vi "theOne.vi"() -> ()   [LabVIEW 2021]
uses:
  <userlib>/er4commlib_labview/er4commlib_labview.lvlib
panel:
  in  "stop":bool
  in  "stop 2":bool
  in  "Boolean":bool
  out "Error String Out":string
  out "error in (no error)":errorcluster
  out "Display 4":dbl[][](graph)
  out "x":dbl
  out "pulseTrainImage":picture
  in  "path to pulseTrainImage file jpg":path=path "C:/neoDiag/MrAnderson/Img/volProtVarAmpl.jpg"
  out "Display 3":dbl[][](graph)=[[0.0, 0.0, 0.0, 0.0, 0.0, 0.0, 0.0, 0.0, 0.0, 0.0, 0.0, 0.0, 0.0, 0.0, 0.0, 0.0, 0.0, 0.0, 0.0, 0.0, 0.0, 0.0, 0.0, 0.0, 0.0, 0.0, 0.0, 0.0, 0.0, 0.0, 0.0, 0.0, 0.0, 0.0, 0.0, 0.0, 0.0, 0.0, 0.0, 0.0, 0.0, 0.0, 0.0, 0.0, 0.0, 0.0, 0.0, 0.0, 0.0, 0.0, 0.0, 0.0, 0.0, 0.0, 0.0, 0.0, 0.0, 0.0, 0.0, 0.0, 0.0, 0.0, 0.0, 0.0, 0.0, 0.0, 0.0, 0.0, 0.0, 0.0, 0.0, 0.0, 0.0, 0.0, 0.0, 0.0, 0.0, 0.0, 0.0, 0.0, 0.0, 0.0, 0.0, 0.0, 0.0, 0.0, 0.0, 0.0, 0.0, 0.0, 0.0, 0.0, 0.0, 0.0, 0.0, 0.0, 0.0, 0.0, 0.0, 0.0, 0.0, 0.0, 0.0, 0.0, 0.0, 0.0, 0.0, 0.0, 0.0, 0.0, 0.0, 0.0, 0.0, 0.0, 0.0, 0.0, 0.0, 0.0, 0.0, 0.0, 0.0, 0.0, 0.0, 0.0, 0.0, 0.0, 0.0, 0.0], [0.004272591326639607, -0.0012207403790398877, -0.008545182653279214, -0.011597033600878933, -0.01281777397991882, -0.013428144169438765, -0.017090365306558428, -0.019531846064638203, -0.01586962492751854, -0.014648884548478652, -0.009765923032319102, -0.007324442274239326, -0.0030518509475997192, 0.004272591326639607, 0.007324442274239326, 0.009765923032319102, 0.013428144169438765, 0.017090365306558428, 0.019531846064638203, 0.02075258644367809, 0.020142216254158147, 0.01770073549607837, 0.014648884548478652, 0.009155552842799158, 0.0061037018951994385, 0.0012207403790398877, -0.003662221137119663, -0.009155552842799158, -0.01098666341135899, -0.01281777397991882, -0.016479995117038484, -0.019531846064638203, -0.017090365306558428, -0.015259254737998596, -0.013428144169438765, -0.00793481246375927, -0.0024414807580797754, 0.0012207403790398877, 0.0061037018951994385, 0.01098666341135899, 0.015259254737998596, 0.016479995117038484, 0.01892147587511826, 0.023194067201757866, 0.02075258644367809, 0.02075258644367809, 0.01586962492751854, 0.01098666341135899, 0.00793481246375927, 0.0012207403790398877, -0.004882961516159551, -0.008545182653279214, -0.01098666341135899, -0.013428144169438765, -0.014648884548478652, -0.018311105685598315, -0.020142216254158147, -0.016479995117038484, -0.013428144169438765, -0.009765923032319102, -0.004882961516159551, -0.0018311105685598315, 0.0030518509475997192, 0.008545182653279214, 0.012207403790398877, 0.01586962492751854, 0.016479995117038484, 0.018311105685598315, 0.020142216254158147, 0.01892147587511826, 0.017090365306558428, 0.013428144169438765, 0.009155552842799158, 0.0061037018951994385, -0.0012207403790398877, -0.0061037018951994385, -0.01098666341135899, -0.014648884548478652, -0.014038514358958708, -0.018311105685598315, -0.020142216254158147, -0.01770073549607837, -0.014648884548478652, -0.012207403790398877, -0.009155552842799158, -0.003662221137119663, 0.0006103701895199438, 0.0061037018951994385, 0.01098666341135899, 0.013428144169438765, 0.015259254737998596, 0.017090365306558428, 0.019531846064638203, 0.018311105685598315, 0.017090365306558428, 0.014648884548478652, 0.009155552842799158, 0.0061037018951994385, 0.0018311105685598315, -0.005493331705679495, -0.008545182653279214, -0.012207403790398877, -0.012207403790398877, -0.014648884548478652, -0.018311105685598315, -0.017090365306558428, -0.016479995117038484, -0.01281777397991882, -0.00793481246375927, -0.005493331705679495, -0.0012207403790398877, 0.0061037018951994385, 0.01098666341135899, 0.014038514358958708, 0.01586962492751854, 0.016479995117038484, 0.019531846064638203, 0.020142216254158147, 0.018311105685598315, 0.014648884548478652, 0.014648884548478652, 0.009155552842799158, 0.003662221137119663, -0.0018311105685598315, -0.00793481246375927, -0.010376293221839045, -0.013428144169438765, -0.015259254737998596], [0.0012207403790398877, -0.003662221137119663, -0.008545182653279214, -0.011597033600878933, -0.014038514358958708, -0.014648884548478652, -0.016479995117038484, -0.01770073549607837, -0.015259254737998596, -0.013428144169438765, -0.011597033600878933, -0.008545182653279214, -0.004882961516159551, 0.0006103701895199438, 0.005493331705679495, 0.007324442274239326, 0.008545182653279214, 0.009765923032319102, 0.012207403790398877, 0.014038514358958708, 0.01281777397991882, 0.01098666341135899, 0.00793481246375927, 0.004882961516159551, 0.0024414807580797754, -0.0024414807580797754, -0.0061037018951994385, -0.010376293221839045, -0.011597033600878933, -0.013428144169438765, -0.014648884548478652, -0.017090365306558428, -0.01586962492751854, -0.014038514358958708, -0.01281777397991882, -0.00793481246375927, -0.005493331705679495, -0.0030518509475997192, 0.0030518509475997192, 0.007324442274239326, 0.009155552842799158, 0.010376293221839045, 0.012207403790398877, 0.015259254737998596, 0.014038514358958708, 0.012207403790398877, 0.009765923032319102, 0.0061037018951994385, 0.0030518509475997192, 0.0006103701895199438, -0.005493331705679495, -0.009155552842799158, -0.01098666341135899, -0.014038514358958708, -0.014038514358958708, -0.017090365306558428, -0.01586962492751854, -0.01586962492751854, -0.012207403790398877, -0.010376293221839045, -0.00793481246375927, -0.004272591326639607, 0.0018311105685598315, 0.005493331705679495, 0.007324442274239326, 0.010376293221839045, 0.012207403790398877, 0.01281777397991882, 0.014648884548478652, 0.013428144169438765, 0.01098666341135899, 0.008545182653279214, 0.005493331705679495, 0.003662221137119663, -0.0030518509475997192, -0.006714072084719382, -0.008545182653279214, -0.01281777397991882, -0.014648884548478652, -0.01586962492751854, -0.01586962492751854, -0.015259254737998596, -0.014648884548478652, -0.01098666341135899, -0.007324442274239326, -0.003662221137119663, -0.0012207403790398877, 0.0024414807580797754, 0.0061037018951994385, 0.009765923032319102, 0.009765923032319102, 0.012207403790398877, 0.015259254737998596, 0.014648884548478652, 0.01098666341135899, 0.009155552842799158, 0.007324442274239326, 0.003662221137119663, 0.0, -0.004882961516159551, -0.009155552842799158, -0.011597033600878933, -0.013428144169438765, -0.014648884548478652, -0.01586962492751854, -0.017090365306558428, -0.016479995117038484, -0.014648884548478652, -0.008545182653279214, -0.005493331705679495, -0.0030518509475997192, 0.0018311105685598315, 0.004882961516159551, 0.008545182653279214, 0.010376293221839045, 0.011597033600878933, 0.014038514358958708, 0.014648884548478652, 0.01281777397991882, 0.009765923032319102, 0.009155552842799158, 0.0061037018951994385, 0.0024414807580797754, -0.0030518509475997192, -0.0061037018951994385, -0.010376293221839045, -0.012207403790398877, -0.012207403790398877], [-0.0061037018951994385, -0.012207403790398877, -0.015259254737998596, -0.018311105685598315, -0.022583697012237922, -0.022583697012237922, -0.023194067201757866, -0.02380443739127781, -0.02380443739127781, -0.022583697012237922, -0.02075258644367809, -0.016479995117038484, -0.013428144169438765, -0.007324442274239326, -0.0024414807580797754, 0.0, 0.0012207403790398877, 0.0012207403790398877, 0.004882961516159551, 0.006714072084719382, 0.003662221137119663, 0.0024414807580797754, 0.0006103701895199438, -0.0018311105685598315, -0.004882961516159551, -0.009155552842799158, -0.014038514358958708, -0.018311105685598315, -0.021362956633198035, -0.022583697012237922, -0.02380443739127781, -0.02685628833887753, -0.02685628833887753, -0.024414807580797754, -0.02197332682271798, -0.017090365306558428, -0.012207403790398877, -0.009155552842799158, -0.003662221137119663, 0.0, 0.0030518509475997192, 0.0030518509475997192, 0.003662221137119663, 0.006714072084719382, 0.006714072084719382, 0.003662221137119663, 0.0030518509475997192, 0.0, -0.003662221137119663, -0.007324442274239326, -0.011597033600878933, -0.015259254737998596, -0.017090365306558428, -0.020142216254158147, -0.021362956633198035, -0.024414807580797754, -0.024414807580797754, -0.023194067201757866, -0.02075258644367809, -0.018311105685598315, -0.01586962492751854, -0.01281777397991882, -0.006714072084719382, -0.0030518509475997192, 0.0006103701895199438, 0.0030518509475997192, 0.0030518509475997192, 0.005493331705679495, 0.0061037018951994385, 0.003662221137119663, 0.003662221137119663, 0.0030518509475997192, -0.0024414807580797754, -0.004882961516159551, -0.009155552842799158, -0.016479995117038484, -0.01892147587511826, -0.02075258644367809, -0.02197332682271798, -0.02380443739127781, -0.026245918149357585, -0.02380443739127781, -0.024414807580797754, -0.02197332682271798, -0.017090365306558428, -0.014038514358958708, -0.008545182653279214, -0.004272591326639607, -0.0012207403790398877, 0.0030518509475997192, 0.003662221137119663, 0.004882961516159551, 0.007324442274239326, 0.0061037018951994385, 0.003662221137119663, 0.0012207403790398877, -0.0012207403790398877, -0.004272591326639607, -0.00793481246375927, -0.01281777397991882, -0.01770073549607837, -0.019531846064638203, -0.020142216254158147, -0.022583697012237922, -0.026245918149357585, -0.024414807580797754, -0.02380443739127781, -0.02197332682271798, -0.01770073549607837, -0.014648884548478652, -0.01281777397991882, -0.0061037018951994385, 0.0006103701895199438, 0.0012207403790398877, 0.0030518509475997192, 0.003662221137119663, 0.006714072084719382, 0.004882961516159551, 0.004882961516159551, 0.0024414807580797754, 0.0, -0.003662221137119663, -0.00793481246375927, -0.012207403790398877, -0.016479995117038484, -0.02075258644367809, -0.021362956633198035, -0.022583697012237922], [-0.004882961516159551, -0.011597033600878933, -0.015259254737998596, -0.01770073549607837, -0.02197332682271798, -0.023194067201757866, -0.026245918149357585, -0.028077028717917417, -0.02685628833887753, -0.02380443739127781, -0.020142216254158147, -0.015259254737998596, -0.010376293221839045, -0.005493331705679495, 0.0024414807580797754, 0.004882961516159551, 0.009155552842799158, 0.009765923032319102, 0.013428144169438765, 0.015259254737998596, 0.012207403790398877, 0.010376293221839045, 0.006714072084719382, 0.0018311105685598315, -0.0012207403790398877, -0.007324442274239326, -0.014648884548478652, -0.01770073549607837, -0.02075258644367809, -0.02075258644367809, -0.02563554795983764, -0.028077028717917417, -0.02563554795983764, -0.025025177770317698, -0.02075258644367809, -0.017090365306558428, -0.01281777397991882, -0.00793481246375927, -0.0018311105685598315, 0.003662221137119663, 0.0061037018951994385, 0.009155552842799158, 0.010376293221839045, 0.01281777397991882, 0.01281777397991882, 0.010376293221839045, 0.007324442274239326, 0.003662221137119663, -0.0006103701895199438, -0.003662221137119663, -0.014038514358958708, -0.01770073549607837, -0.019531846064638203, -0.024414807580797754, -0.024414807580797754, -0.028077028717917417, -0.028077028717917417, -0.02685628833887753, -0.023194067201757866, -0.01892147587511826, -0.015259254737998596, -0.011597033600878933, -0.0030518509475997192, 0.0012207403790398877, 0.003662221137119663, 0.00793481246375927, 0.009155552842799158, 0.013428144169438765, 0.014038514358958708, 0.011597033600878933, 0.00793481246375927, 0.0061037018951994385, 0.0012207403790398877, -0.0018311105685598315, -0.006714072084719382, -0.013428144169438765, -0.017090365306558428, -0.022583697012237922, -0.023194067201757866, -0.02563554795983764, -0.02868739890743736, -0.024414807580797754, -0.022583697012237922, -0.020142216254158147, -0.014648884548478652, -0.014038514358958708, -0.006714072084719382, 0.0, 0.003662221137119663, 0.0061037018951994385, 0.008545182653279214, 0.012207403790398877, 0.014038514358958708, 0.013428144169438765, 0.012207403790398877, 0.00793481246375927, 0.003662221137119663, -0.0006103701895199438, -0.005493331705679495, -0.012207403790398877, -0.018311105685598315, -0.021362956633198035, -0.023194067201757866, -0.02685628833887753, -0.02868739890743736, -0.027466658528397473, -0.02563554795983764, -0.022583697012237922, -0.018311105685598315, -0.014038514358958708, -0.010376293221839045, -0.003662221137119663, 0.0024414807580797754, 0.005493331705679495, 0.00793481246375927, 0.008545182653279214, 0.013428144169438765, 0.01281777397991882, 0.01098666341135899, 0.01098666341135899, 0.005493331705679495, 0.0006103701895199438, -0.0018311105685598315, -0.009765923032319102, -0.01586962492751854, -0.01892147587511826, -0.02197332682271798, -0.02197332682271798], [0.0, 0.0, 0.0, 0.0, 0.0, 0.0, 0.0, 0.0, 0.0, 0.0, 0.0, 0.0, 0.0, 0.0, 0.0, 0.0, 0.0, 0.0, 0.0, 0.0, 0.0, 0.0, 0.0, 0.0, 0.0, 0.0, 0.0, 0.0, 0.0, 0.0, 0.0, 0.0, 0.0, 0.0, 0.0, 0.0, 0.0, 0.0, 0.0, 0.0, 0.0, 0.0, 0.0, 0.0, 0.0, 0.0, 0.0, 0.0, 0.0, 0.0, 0.0, 0.0, 0.0, 0.0, 0.0, 0.0, 0.0, 0.0, 0.0, 0.0, 0.0, 0.0, 0.0, 0.0, 0.0, 0.0, 0.0, 0.0, 0.0, 0.0, 0.0, 0.0, 0.0, 0.0, 0.0, 0.0, 0.0, 0.0, 0.0, 0.0, 0.0, 0.0, 0.0, 0.0, 0.0, 0.0, 0.0, 0.0, 0.0, 0.0, 0.0, 0.0, 0.0, 0.0, 0.0, 0.0, 0.0, 0.0, 0.0, 0.0, 0.0, 0.0, 0.0, 0.0, 0.0, 0.0, 0.0, 0.0, 0.0, 0.0, 0.0, 0.0, 0.0, 0.0, 0.0, 0.0, 0.0, 0.0, 0.0, 0.0, 0.0, 0.0, 0.0, 0.0, 0.0, 0.0, 0.0, 0.0]]
  out "counterArraySize":i32=2500
  out "runningCounterFlag":bool=TRUE
  out "runningCounter":i32=1488
  out "initialized array":dbl[][](array[numeric])
  out "function return":u32(ring)
  in  "Tab Control":enum32{"AcqPara", "AdvPara"}(tab)
  in  "Acquisition Parameters":T1={"Camera "=FALSE, "Voltage stimulus"=FALSE, "Period [ms]"=200.0, "Duration [ms]"=0.2, "Delay [ms]"=0.0, "Pulses [#]"=10, "Vhold [mV]"=-50.0, "Vpulse [mV]"=0.0, "Vstep [mV]"=10.0, "N"=10, "Thold [ms]"=0.0, "Tpulse [ms]"=200.0, "sampling rate [kHz]"="1,25", "current range [nA]"="20", "time [s]"=2.0} {"Tpulse [ms]" format="%_5f"; "Thold [ms]" format="%_5f"; "Vstep [mV]" format="%_5f"; "Vpulse [mV]" format="%_5f"; "Vhold [mV]" format="%_5f"; "Delay [ms]" format="%_5f"; "Duration [ms]" format="%_5f"; "Period [ms]" format="%_5f"}
  in  "advancedSettings":T2={"Channels to read"=6, "update rate of main loop"=100}
  out "Error Out Int":u32
  out "Error Out String":string
  out "E4 parameters":T3={"currentChannelsNum out"=1, "voltageChannelsNum out"=4, "gpChannelsNum out"=1, "sampling rate [kHz]"=1.25, "real sampling rate [kHz]"=1.220703125, "Ch_min"=-20.0, "Ch_max"=20.0, "Ch_step"=0.0006103701895199438, "Ch_unit"=1e-09}
  in  "Display 1":cluster{"ChArray":bool[]}={"ChArray"=[FALSE, TRUE, TRUE, TRUE, FALSE, FALSE]}
  out "Display 2":dbl[][](graph)
  in  "Live":bool
  out "status out":T4={"availableDataPackets"=128, "bufferOverflowFlag"=FALSE, "lostDataFlag"=FALSE, "saturationFlag"=FALSE, "currentRangeIncreaseFlag"=FALSE, "currentRangeDecreaseFlag"=TRUE, "communicationErrorFlag"=FALSE}
  out "Error Read":errorcluster
  # "DataCh1"
  # "DataCh2"
  # "DataCh3"
  # "DataCh4"
  # "Voltage"
  # "Trigger"
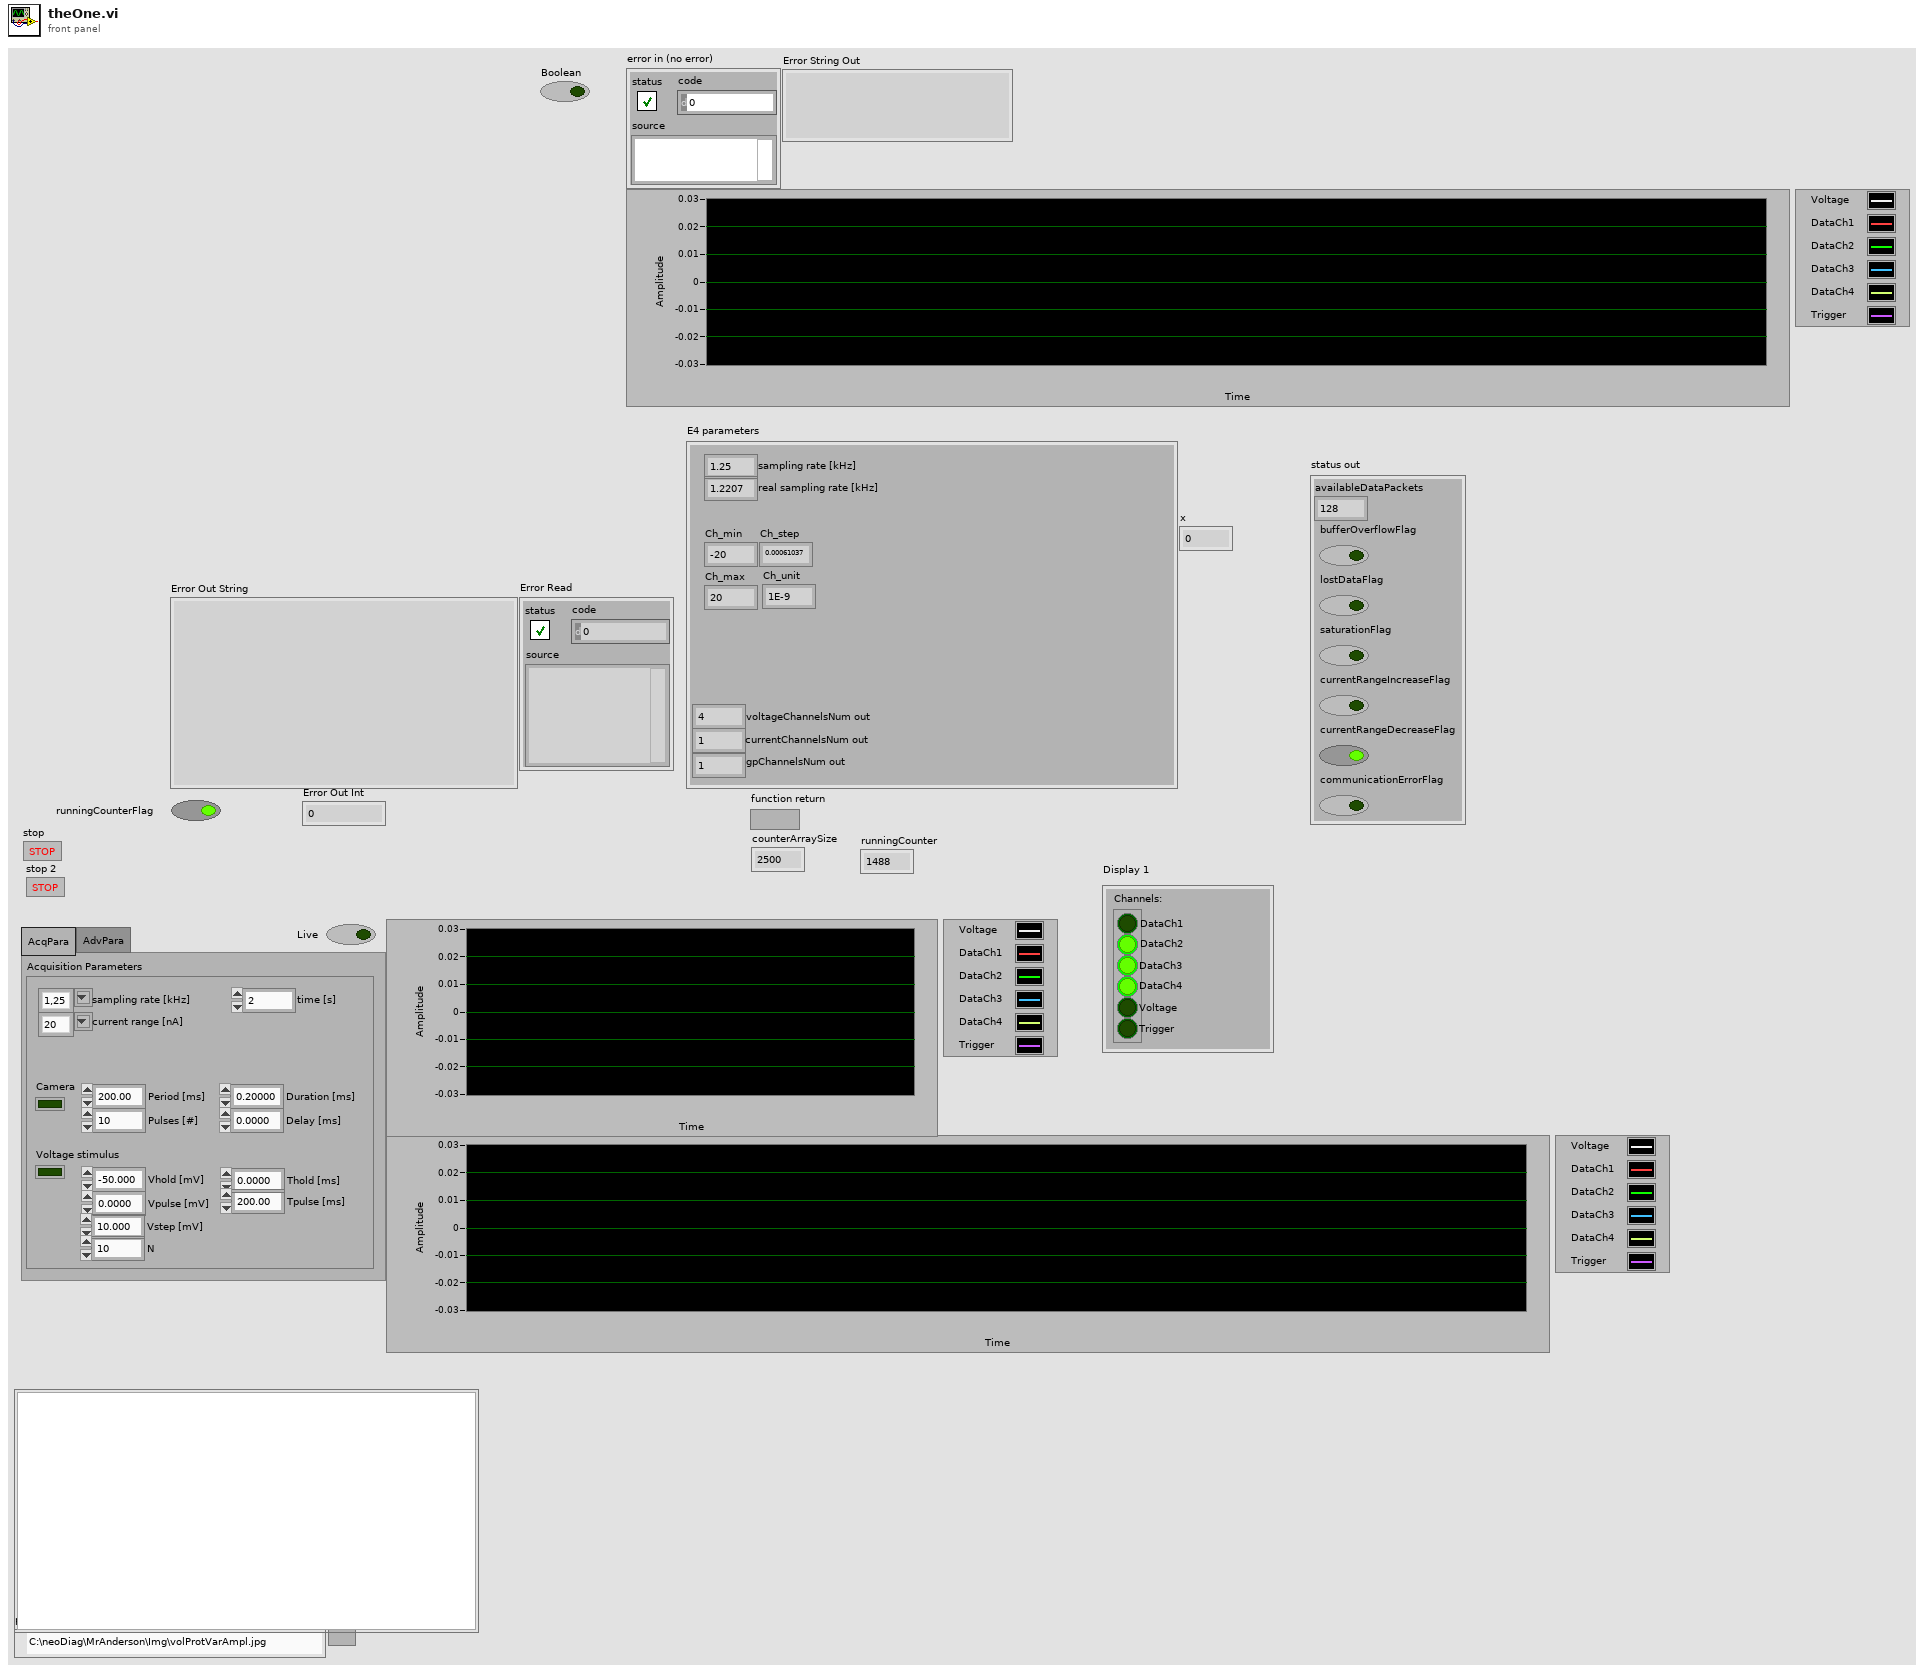
[diagram p1: front panel]
types:
  T1 = cluster{"Camera ":bool, "Voltage stimulus":bool, "Period [ms]":dbl, "Duration [ms]":dbl, "Delay [ms]":dbl, "Pulses [#]":u32, "Vhold [mV]":dbl, "Vpulse [mV]":dbl, "Vstep [mV]":dbl, "N":u32, "Thold [ms]":dbl, "Tpulse [ms]":dbl, "sampling rate [kHz]":string, "current range [nA]":string, "time [s]":dbl}
  T2 = cluster{"Channels to read":i32, "update rate of main loop":i32}
  T3 = cluster{"currentChannelsNum out":u32, "voltageChannelsNum out":u32, "gpChannelsNum out":u32, "sampling rate [kHz]":dbl, "real sampling rate [kHz]":dbl, "Ch_min":dbl, "Ch_max":dbl, "Ch_step":dbl, "Ch_unit":dbl}
  T4 = cluster{"availableDataPackets":u32, "bufferOverflowFlag":bool, "lostDataFlag":bool, "saturationFlag":bool, "currentRangeIncreaseFlag":bool, "currentRangeDecreaseFlag":bool, "communicationErrorFlag":bool}
  T5 = typedef "imagedata.ctl" = cluster{"image type":i32, "image depth":i32, "image":u8[], "mask":u8[], "colors":u32[], "Rectangle":cluster{"left":i16, "top":i16, "right":i16, "bottom":i16}}
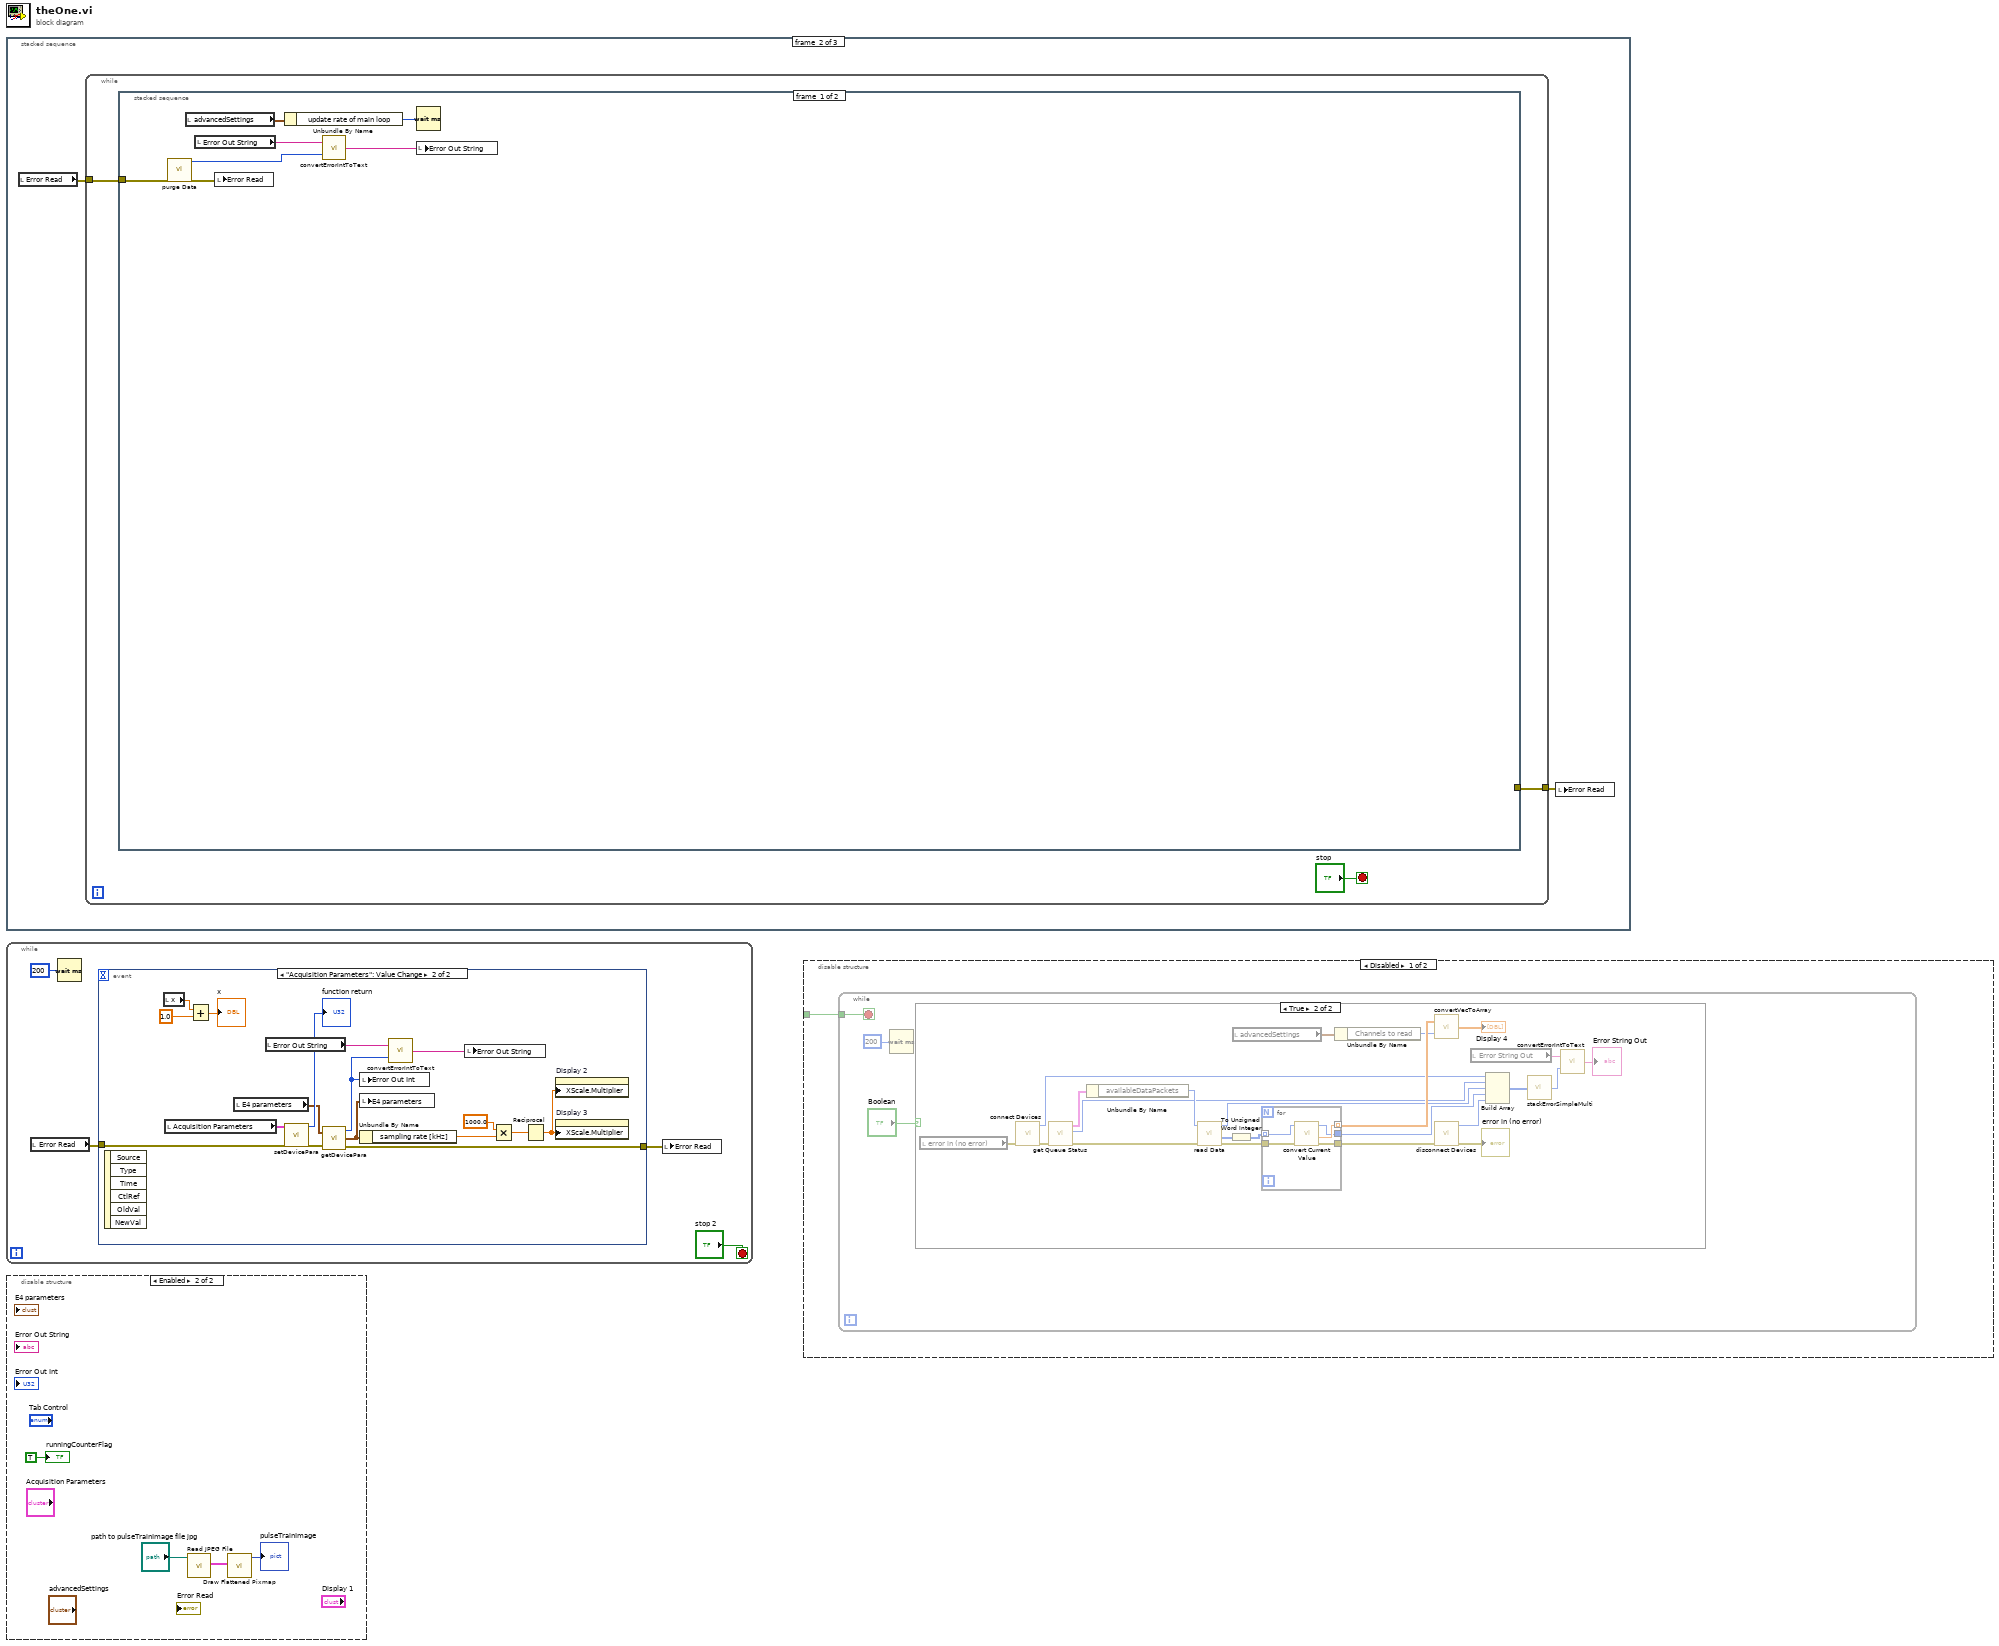
[diagram p0: block diagram]
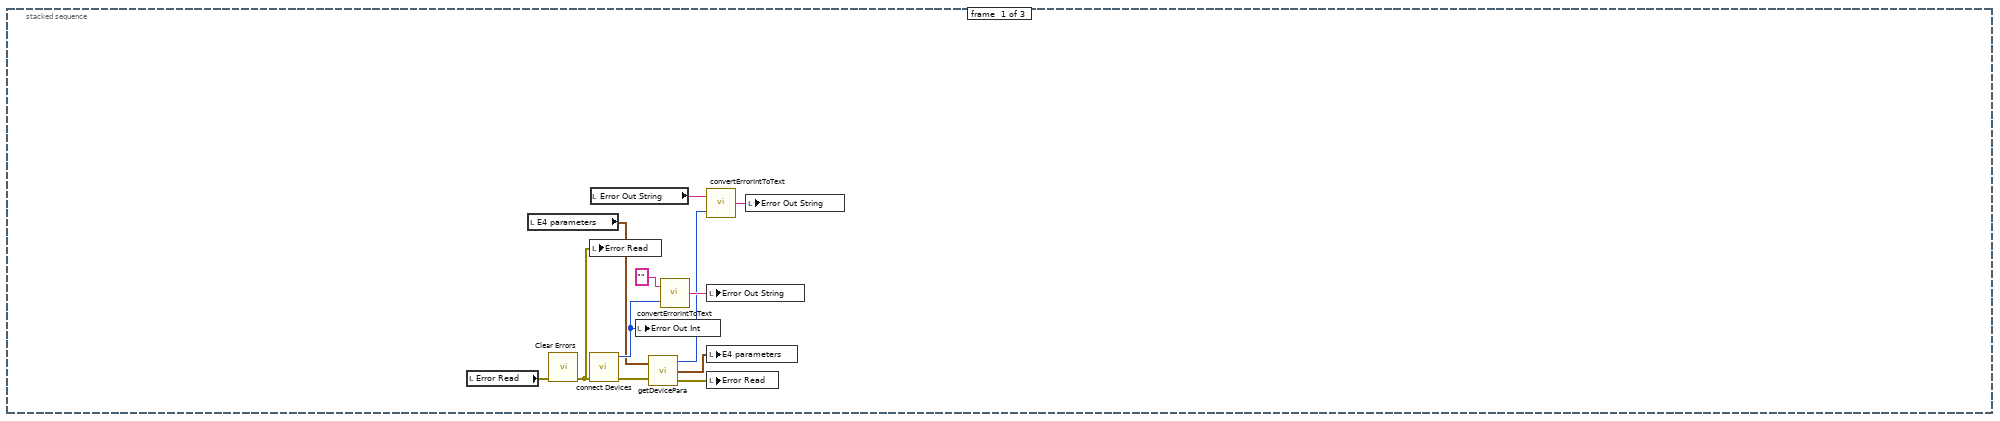
[diagram p4: hidden frame]
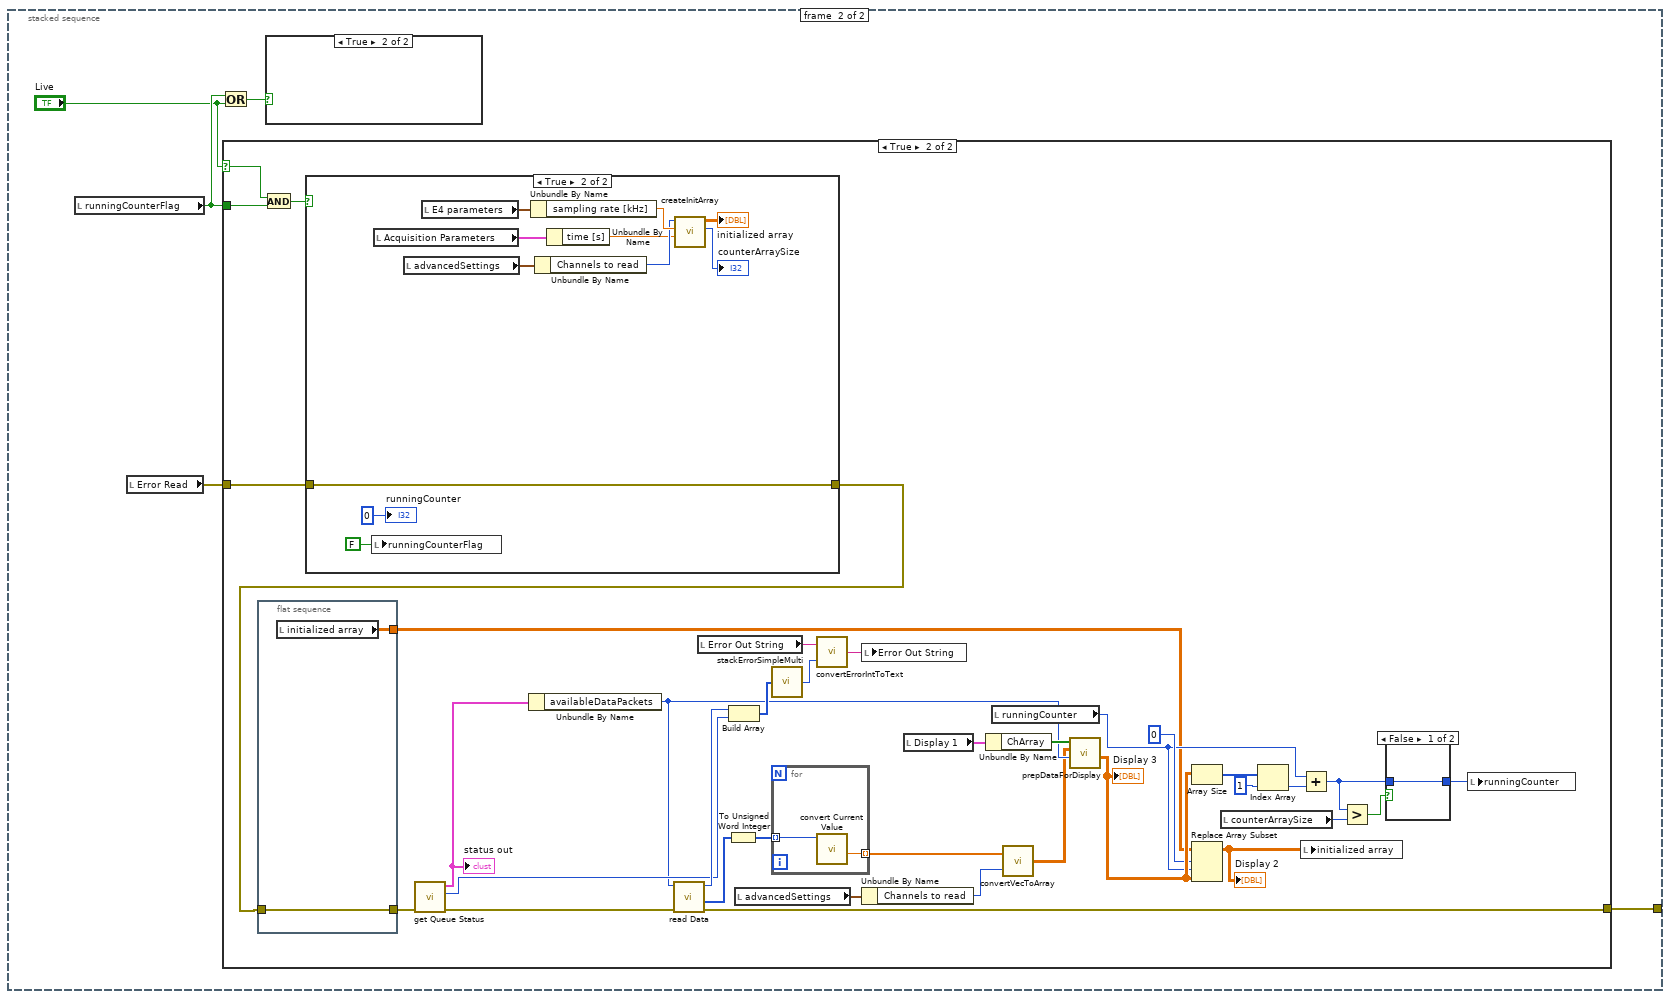
[diagram p5: hidden frame]
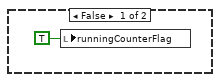
[diagram p6: hidden frame]
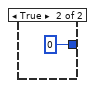
[diagram p9: hidden frame]
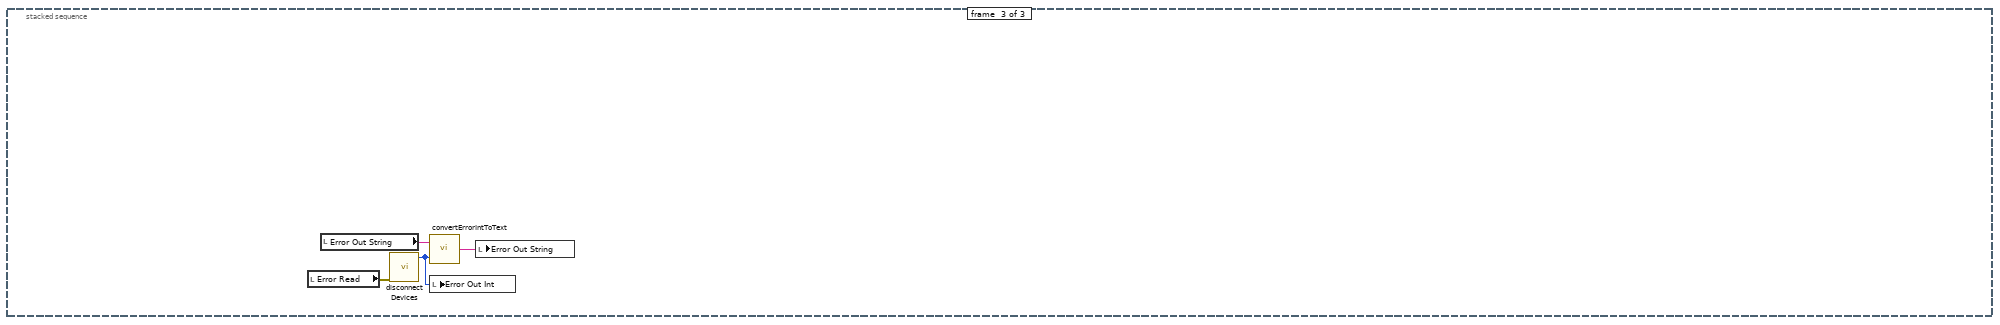
[diagram p10: hidden frame]
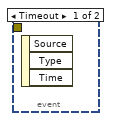
[diagram p11: hidden frame]
diagram:
  n1 = stacked-sequence {
    frame #0 {
      n2 = local read "Error Read"() -> (w3:errorcluster)
      n3 = local read "E4 parameters"() -> (w8:T3)
      n4 = call <vilib>:"Clear Errors.vi"("error in (no error)"=w3) -> ("error out"=w2:errorcluster)  [unwired: 5 in, 1 out]
      n5 = local write "Error Read"(w2) -> ()
      n6 = call <userlib>:"connect Devices.vi"("error in (no error)"=w2) -> ("error out"=w9:errorcluster, "function return"=w12:u32)  [unwired: 9 in]
      n7 = local read "Error Out String"() -> (w5:string)
      n8 = local write "Error Out Int"(w12) -> ()
      n9 = call "getDevicePara.vi"("Seetings in"=w8, "error in (no error)"=w9) -> ("Error Out"=w6:u32, "Seetings out"=w7:T3, "error out"=w1:errorcluster)
      n10 = call "convertErrorIntToText.vi"("Error Int In (function return)"=w12, "Error String In"="" ("String 2")) -> ("Error String Out"=w11:string)
      n11 = call "convertErrorIntToText.vi"("Error Int In (function return)"=w6, "Error String In"=w5) -> ("Error String Out"=w4:string)
      n12 = local write "Error Out String"(w11) -> ()
      n13 = local write "E4 parameters"(w7) -> ()
      n14 = local write "Error Read"(w1) -> ()
      n15 = local write "Error Out String"(w4) -> ()
    }
    frame #1 {
      n16 = local read "Error Read"() -> (w13:errorcluster)
      n17 = while {
        tunnel: w13 -> [w16]
        tunnel: [w17] -> w14
        stop <- "stop" stop-if-true
        n18 = stacked-sequence {
          tunnel: w16 -> [w24 _]
          tunnel: [_ w29] -> w17
          frame #0 {
            n19 = call <userlib>:"purge Data.vi"("error in (no error)"=w24) -> ("error out"=w18:errorcluster, "function return"=w22:u32)  [unwired: 9 in]
            n20 = local read "advancedSettings"() -> (w20:T2)
            n21 = local read "Error Out String"() -> (w23:string)
            n22 = local write "Error Read"(w18) -> ()
            n23 = Unbundle By Name(w20) -> ("update rate of main loop"=w19:i32)
            n24 = call "convertErrorIntToText.vi"("Error Int In (function return)"=w22, "Error String In"=w23) -> ("Error String Out"=w21:string)
            n25 = Wait (ms)(milliseconds to wait=w19) -> ()  [unwired: 1 out]
            n26 = local write "Error Out String"(w21) -> ()
          }
          frame #1 {
            n27 = local read "runningCounterFlag"() -> (w28:bool)
            n28 = local read "Error Read"() -> (w25:errorcluster)
            n29 = Or(x=w28, y="Live") -> (x .or. y?=w26:bool)
            n30 = case shown="True" "Live" {
              selector: "Live" -> [_ w45]
              tunnel: w25 -> [w31 w41]
              tunnel: [w31 w65] -> w29
              tunnel: w28 -> [_ w44]
              frame False {
              }
              frame True {
                n31 = flat-sequence {
                  tunnel: w32 -> [w69]
                  tunnel: [w69] -> w34
                  tunnel: [w68] -> w35
                  frame #0 {
                    n32 = local read "initialized array"() -> (w68:dbl[][])
                  }
                }
                n33 = And(x=w45, y=w44) -> (x .and. y?=w43:bool)
                n34 = case shown="True" w43 {
                  tunnel: w41 -> [w70 w73]
                  tunnel: [w70 w73] -> w32
                  frame False {
                  }
                  frame True {
                    n35 = local write "runningCounterFlag"(FALSE ("runningCounterFlag")) -> ()
                    n36 = local read "Acquisition Parameters"() -> (w72:T1)
                    n37 = local read "advancedSettings"() -> (w76:T2)
                    n38 = local read "E4 parameters"() -> (w78:T3)
                    n39 = Unbundle By Name(w78) -> ("sampling rate [kHz]"=w79:dbl)
                    n40 = Unbundle By Name(w76) -> ("Channels to read"=w77:i32)
                    n41 = Unbundle By Name(w72) -> ("time [s]"=w71:dbl)
                    n42 = call "createInitArray.vi"("timeAxisLim"=w71, "sampling rate [kHz]"=w79, "Channels to read"=w77) -> ("Numeric"=→"counterArraySize":i32, "Array"=→"initialized array":dbl[][])  [unwired: 7 in]
                    "runningCounter" <- 0 ("runningCounter")
                  }
                }
                n43 = call <userlib>:"get Queue Status.vi"("error in (no error)"=w34) -> ("error out"=w66:errorcluster, "function return"=w63:u32, "status out"=w67:T4)  [unwired: 8 in]
                "status out" <- w67
                n44 = Unbundle By Name(w67) -> ("availableDataPackets"=w55:u32)
                n45 = call <userlib>:"read Data.vi"("error in (no error)"=w66, "dataToRead"=w55) -> ("error out"=w65:errorcluster, "buffer out"=w33:i16[], "function return"=w64:u32)  [unwired: 6 in, 1 out]
                n46 = local read "Error Out String"() -> (w59:string)
                n47 = To Unsigned Word Integer(number=w33) -> (unsigned 16bit integer=w54:u16[])
                n48 = Build Array(w64, w63) -> (w62:u32[])
                n49 = local read "advancedSettings"() -> (w56:T2)
                n50 = call "stackErrorSimpleMulti.vi"("Error List"=w62) -> ("Error Out"=w61:u32)
                n51 = for {
                  tunnel: w54 -> [w85] mode=indexing
                  tunnel: [w84] -> w53 mode=indexing
                  n52 = call <userlib>:"convert Current Value.vi"("intValue"=w85) -> ("fltValue out"=w84:dbl)  [unwired: 8 in, 2 out]
                }
                n53 = call "convertErrorIntToText.vi"("Error Int In (function return)"=w61, "Error String In"=w59) -> ("Error String Out"=w60:string)
                n54 = local write "Error Out String"(w60) -> ()
                n55 = Unbundle By Name(w56) -> ("Channels to read"=w52:i32)
                n56 = local read "Display 1"() -> (w58:cluster{"ChArray":bool[]})
                n57 = Unbundle By Name(w58) -> ("ChArray"=w57:bool[])
                n58 = local read "runningCounter"() -> (w37:i32)
                n59 = call "convertVecToArray.vi"("Channels"=w52, "buffer in"=w53) -> ("Array"=w40:dbl[][])
                n60 = call "prepDataForDisplay.vi"("dataToRead"=w55, "Array in"=w40, "ChArray"=w57) -> ("AllChOut"=w39:dbl[][])  [unwired: 6 in, 2 out]
                "Display 3" <- w39
                n61 = Array Size(array=w39) -> (size(s)=w51:i32[])
                n62 = Replace Array Subset(array=w35, new element=w39, index (row)=0 ("disabled index (row)"), index (col)=w37) -> (w36:dbl[][])
                "Display 2" <- w36
                n63 = local read "counterArraySize"() -> (w42:i32)
                n64 = Index Array(array=w51, index=1) -> (element=w49:i32)
                n65 = Add(x=w37, y=w49) -> (x+y=w47:i32)
                n66 = local write "initialized array"(w36) -> ()
                n67 = Greater?(x=w47, y=w42) -> (0:w48:bool)
                n68 = case shown="False" w48 {
                  tunnel: w47 -> [w82 _]
                  tunnel: [w82 0] -> w46
                  frame False {
                  }
                  frame True {
                  }
                }
                n69 = local write "runningCounter"(w46) -> ()
              }
            }
            n70 = case shown="True" w26 {
              frame False {
                n71 = local write "runningCounterFlag"(TRUE ("runningCounterFlag")) -> ()
              }
              frame True {
              }
            }
          }
        }
      }
      n72 = local write "Error Read"(w14) -> ()
    }
    frame #2 {
      n73 = local read "Error Read"() -> (w86:errorcluster)
      n74 = local read "Error Out String"() -> (w89:string)
      n75 = call <userlib>:"disconnect Devices.vi"("error in (no error)"=w86) -> ("function return"=w88:u32)  [unwired: 9 in, 1 out]
      n76 = call "convertErrorIntToText.vi"("Error Int In (function return)"=w88, "Error String In"=w89) -> ("Error String Out"=w87:string)
      n77 = local write "Error Out Int"(w88) -> ()
      n78 = local write "Error Out String"(w87) -> ()
    }
  }
  n79 = while {
    stop <- "stop 2" stop-if-true
    n80 = local read "Error Read"() -> (w91:errorcluster)
    n81 = Wait (ms)(milliseconds to wait=u32 200) -> ()  [unwired: 1 out]
    n82 = event shown="[1] \"Acquisition Parameters\": Value Change" {
      selector: _ -> [_ _]
      dyn-events: _ -> [_ _]
      timeout: _ -> [_ _]
      tunnel: [_ w95] -> w92
      tunnel: w91 -> [_ w94]
      event Timeout {
        n83 = event-data() -> ()  [unwired: 1 in, 3 out]
      }
      event "Acquisition Parameters": Value Change {
        n84 = event-data() -> ()  [unwired: 1 in, 6 out]
        n85 = local read "x"() -> (w109:dbl)
        n86 = local read "Acquisition Parameters"() -> (w102:T1)
        n87 = Add(x=w109, y=1.0) -> (x+y=→"x":dbl)
        n88 = local read "E4 parameters"() -> (w97:T3)
        n89 = local read "Error Out String"() -> (w99:string)
        n90 = call "setDevicePara.vi"("error in (no error)"=w94, "Acquisition Parameters 2"=w102) -> ("error out"=w103:errorcluster, "function return"=→"function return":u32)  [unwired: 8 in]
        n91 = call "getDevicePara.vi"("Seetings in"=w97, "error in (no error)"=w103) -> ("Error Out"=w100:u32, "Seetings out"=w101:T3, "error out"=w95:errorcluster)
        n92 = local write "Error Out Int"(w100) -> ()
        n93 = local write "E4 parameters"(w101) -> ()
        n94 = Unbundle By Name(w101) -> ("sampling rate [kHz]"=w106:dbl)
        n95 = call "convertErrorIntToText.vi"("Error Int In (function return)"=w100, "Error String In"=w99) -> ("Error String Out"=w98:string)
        n96 = local write "Error Out String"(w98) -> ()
        n97 = Multiply(x=1000.0, y=w106) -> (x*y=w105:dbl)
        n98 = Reciprocal(x=w105) -> (1/x=w107:dbl)
        n99 = property on="Display 2" class="WFGraph (strict)"("XScale.Multiplier"=w107) -> ()  [unwired: 2 in, 2 out]
        n100 = property on="Display 3" class="WFGraph (strict)"("XScale.Multiplier"=w107) -> ()  [unwired: 2 in, 2 out]
      }
    }
    n101 = local write "Error Read"(w92) -> ()
  }
  n102 = disable-structure shown="Enabled" {
    frame Disabled {
    }
    frame Enabled {
      n103 = call <vilib>:"Read JPEG File.vi"("path to JPEG file"="path to pulseTrainImage file jpg") -> ("image data"=w112:T5)  [unwired: 8 in, 2 out]
      n104 = call <vilib>:"Draw Flattened Pixmap.vi"("image data"=w112) -> ("new picture"=→"pulseTrainImage":picture)  [unwired: 8 in]
      "runningCounterFlag" <- TRUE ("runningCounterFlag")
    }
  }
  n105 = disable-structure shown="Disabled" {
    disable-tunnel: _ -> [w115 _]
    frame Disabled {
      n106 = while {
        tunnel: w115 -> [w117]
        stop <- w117 stop-if-true
        n107 = Wait (ms)(milliseconds to wait=u32 200) -> ()  [unwired: 1 out]
        n108 = case shown="True" "Boolean" {
          frame False {
          }
          frame True {
            n109 = local read "error in (no error)"() -> (w126:errorcluster)
            n110 = call <userlib>:"connect Devices.vi"("error in (no error)"=w126) -> ("error out"=w125:errorcluster, "function return"=w124:u32)  [unwired: 9 in]
            n111 = call <userlib>:"get Queue Status.vi"("error in (no error)"=w125) -> ("error out"=w137:errorcluster, "function return"=w132:u32, "status out"=w141:T4)  [unwired: 8 in]
            n112 = Unbundle By Name(w141) -> ("availableDataPackets"=w140:u32)
            n113 = call <userlib>:"read Data.vi"("error in (no error)"=w137, "dataToRead"=w140) -> ("error out"=w123:errorcluster, "buffer out"=w138:i16[], "function return"=w131:u32)  [unwired: 6 in, 1 out]
            n114 = To Unsigned Word Integer(number=w138) -> (unsigned 16bit integer=w139:u16[])
            n115 = local read "advancedSettings"() -> (w133:T2)
            n116 = for {
              tunnel: w139 -> [w146] mode=indexing
              tunnel: [w145] -> w136 mode=indexing
              tunnel: [w144] -> w120
              tunnel: w123 -> [w143]
              tunnel: [w142] -> w122
              n117 = call <userlib>:"convert Current Value.vi"("error in (no error)"=w143, "intValue"=w146) -> ("error out"=w142:errorcluster, "fltValue out"=w145:dbl, "function return"=w144:u32)  [unwired: 7 in]
            }
            n118 = Unbundle By Name(w133) -> ("Channels to read"=w135:i32)
            n119 = call "convertVecToArray.vi"("Channels"=w135, "buffer in"=w136) -> ("Array"=→"Display 4":dbl[][])
            n120 = call <userlib>:"disconnect Devices.vi"("error in (no error)"=w122) -> ("error out"=→"error in (no error)":errorcluster, "function return"=w119:u32)  [unwired: 9 in]
            n121 = local read "Error String Out"() -> (w127:string)
            n122 = Build Array(w124, w132, w131, w120, w119) -> (w130:u32[])
            n123 = call "stackErrorSimpleMulti.vi"("Error List"=w130) -> ("Error Out"=w129:u32)
            n124 = call "convertErrorIntToText.vi"("Error Int In (function return)"=w129, "Error String In"=w127) -> ("Error String Out"=→"Error String Out":string)
          }
        }
      }
    }
    frame Enabled {
    }
  }
